vi "Parse Message.vi"(1 "Update Message":T2={"Update Command"=enum."Update Switch", "Channel"=0, "Value"=variant}) -> (5 "Update Command":T1=enum."Update Power", 7 "Channel":u8, 8 "Value":variant)   [LabVIEW 2019, in "UI.lvlib"]
uses:
  UI.lvlib
  Update Message.ctl
  Update Command.ctl
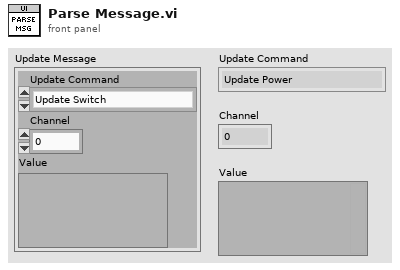
[diagram p1: front panel]
types:
  T1 = typedef "UI.lvlib/Update Command.ctl" = enum16{"Update Frequency", "Update Power", "Update Switch", "Error", "Stop"}
  T2 = typedef "UI.lvlib/Update Message.ctl" = cluster{"Update Command":T1, "Channel":u8, "Value":variant}
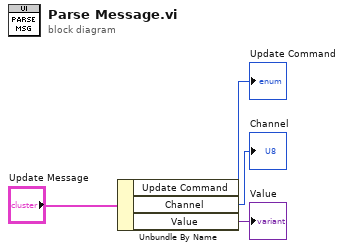
[diagram p0: block diagram]
diagram:
  n1 = Unbundle By Name("Update Message") -> ("Update Command"=→"Update Command":T1, "Channel"=→"Channel":u8, "Value"=→"Value":variant)
